vi "Studienarbeit-Luis-Waldhauser-2023.vi"(8 "error in (no error)":errorcluster) -> (0 "error out":errorcluster)   [LabVIEW 2023]
doc: "Technische Hochschule Nürnberg Georg-Simon Ohm\nAbschlußprüfungen Sommersemester 2021 \nOnline (MS-Teams, 13.3.2021 10.00 Uhr - 15.00 Uhr)\nPrüfer: Herbert Pichlik \nZweitkorrektor: Prof. Dr. Michael Chowanetz\n\nNachname: Müller\nVorname: Stefan\nMatrikelnummer: 08154711\n\nHiermit nehme verbindlich an folgenden Prüfungen teil:\n\nWahlpflichtfach: 080efi:WPF:EFI:0 Titel: LabVIEW und Virtuelle Instrumente\n\nWahlfach: 1010:WF:EFI:0 Titel: LabVIEW Vertiefung"
uses:
  <vilib>/Utility/error.llb/DialogType.ctl
  Users/luisw/Downloads/Studiarbeit/Studiarbeit/state.ctl
  <vilib>/event_ctls.llb/eventvkey.ctl
  <vilib>/Utility/NIReport.llb/Report Type.ctl
  <vilib>/Analysis/baseanly.llb/Mean (DBL).vi
  <vilib>/measure/matone.llb/Harmonic Distortion Analyzer 1 Chan.vi
  <vilib>/measure/maspectr.llb/FFT Power Spectrum and PSD for 1 Chan.vi
  <vilib>/printing/OpenHTMLReport.llb/Open HTML Report in Browser (Path).vi
  <vilib>/Utility/NIReport.llb/NI_report.lvclass
  <vilib>/Utility/NIReport.llb/NI_ReportGenerationCore.lvlib
  <vilib>/measure/NI_MABase.lvlib
  <vilib>/measure/NI_MAPro.lvlib
  <vilib>/Analysis/NI_AALBase.lvlib
panel:
  out "path out":path
  out "Time":string="09:57:22"
  out "Date":string="12.03.2021"
  in  "Tab Control":enum32{"GUI", "Input", "Hidden", "Admin"}(tab)
  out "Sequence Comment":string
  out "Name":string
  out "Seq Measurement":T1(array[cluster])
  in  "Load Sequence":path=path "C:/Program Files/National Instruments/LabVIEW 2020/user.lib/SoSe2021/Sequence-01.xlsx"
  out "FFT":cluster{"f0":dbl, "df":dbl, "magnitude":dbl[]}(graph)={"f0"=0.0, "df"=1.0, "magnitude"=[2.6327073338101692e-05, 4.327304114792483e-05, 1.5673481931988e-05, 0.00025407252568578504, 0.0006345873730570163, 0.001098990914477157, 0.0008159585478017789, 1.2611184277899417, 5.146224925426655, 1.3095648931593402, 2.63970380788412e-05, 0.0006386317455637907, 0.0012590716223286752, 0.0005410344712417312, 0.0001693664822519534, 0.0004908339259456577, 0.0011777334761568917, 0.00037163963536089004, 3.021983314851664e-05, 0.00017377346672736057, 0.0003762593897253986, 0.00023256570049066358, 0.00012724272038241313, 0.000178513498907416, 0.00021924620032822906, 0.0001544896302861912, 8.457623674491461e-06, 5.403062950323495e-05, 0.0001296238557588327, 0.00016495018928055702, 0.0003034184772940682, 0.00015646022009288462, 0.00031162575785944626, 0.0012565613166387428, 0.0006107618849779327, 7.515890864872665e-06, 0.0001419118218565884, 8.036975874934862e-05, 8.488687318252203e-05, 2.5141530202907425e-05, 2.673290688424461e-05, 0.00018239018640602903, 0.0005477270664906835, 0.0014690375427782237, 0.0005559107924960337, 8.301140037468495e-05, 0.00012101523160707916, 0.0008051848168213473, 0.0006343845922274333, 1.3569945226961809e-05, 0.0002627792110390153, 0.0002406122221775621, 0.0002163088212400089, 0.0005756861353742484, 0.0006540662987181892, 0.0005760057147609353, 0.001168214064104931, 0.0009142393249436326, 3.7459985637611555e-05, 6.58826949190464e-05, 0.0003019406937540107, 0.00018554779716880925, 9.112019612896804e-05, 0.0002658304606239494, 0.0005842272847474148, 0.001822778790135895, 0.0020011462573474594, 0.000770952197268878, 0.0003802029039891558, 2.1515126635341356e-05, 8.549323495065751e-05, 4.6310151827152625e-05, 9.24162402997269e-05, 7.024420564693392e-05, 0.00020170519648798685, 0.0008603793021965292, 0.0008822311938917643, 0.001716853456240963, 0.00039036674041830654, 0.0006307930109717719, 0.002044627565204085, 0.0011767234719083748, 0.00020159725845851647, 7.759760038327143e-05, 0.0007509384980458659, 0.0002221474003132149, 0.00016765791243669574, 6.896494488849775e-05, 2.992435621102185e-05, 0.0001591877555499712, 0.0006627411738638841, 0.0006823777206984923, 0.00015280161807136624, 4.9723659888706556e-05, 0.00015953763055465215, 0.00021839526016487058, 6.904122739035353e-05, 0.0003228624565004558, 0.0008641263395326468, 0.0004885756306196472, 5.5452575762701354e-05, 6.667888896910418e-05, 0.00016195387231479331, 0.0005157262849646858, 0.00018487779477048604, 0.0005163607105677836, 0.0008405910681775814, 9.914286246284125e-05, 0.0003983930841559924, 0.0006755226388984388, 1.557357874689003e-05, 3.5271995415016136e-06, 0.00011873017943008137, 0.0001178216082098147, 0.0003321531164868442, 0.0002823966252785709, 0.0001271820869068118, 0.00015734413774907115, 0.00011336787749456681, 0.00030849395695113554, 0.0012548186928315786, 0.0009022685720360012, 5.297998902547502e-05, 2.3303881834746823e-05, 0.00022979277121929284, 9.992147446179476e-05, 0.00014219787549692135, 0.00036985584741512086, 0.0005451942969393532, 0.00022508503372422933, 0.0010284913682260671, 0.0013684067307147309, 0.0004522588358697734, 0.0002703600366179861, 5.5588453885048256e-05, 1.587439002785841e-05, 0.00011966475460832903, 0.00010662390359710843, 9.529947631894765e-05, 9.900928679592479e-05, 0.0007085109743305238, 0.00020493016828895114, 3.9234127841945937e-05, 5.8382921609386196e-05, 6.74673457346776e-05, 3.1706979194275405e-05, 5.5114477174054164e-05, 4.1244190248820976e-05, 8.318994464694256e-05, 0.00021409167282633557, 7.076373237749193e-05, 0.0004444126722076365, 1.4431314640259825e-05, 0.0003017498107005694, 0.00019778188880576763, 0.0004790860486344645, 0.0006681849923944, 0.0005240711139280371, 0.0002346300453842311, 0.0002079119924688067, 0.00014490709524552807, 0.00013212635076267408, 9.022508495594329e-05, 0.000330333713353353, 4.280470532497084e-06, 0.00010134846466738688, 2.400909755508234e-05, 0.00010985927008078305, 0.0003929981111498782, 0.0005400793749820781, 0.0004520034503300079, 9.17009482877119e-05, 0.00011737238653380866, 0.00010319090589896972, 1.6439537841938072e-06, 0.0001283612831574683, 0.00028905567066825236, 0.00021147750147839086, 2.04220484868536e-05, 8.465208277084334e-05, 3.623808768161366e-05, 0.0003773213469952989, 0.00012937830574505138, 0.0003866640298215692, 7.132733306923889e-05, 5.2771987655576355e-05, 5.4455648893278534e-06, 5.582730151819657e-05, 0.00014251337916616028, 0.000289780881654889, 0.0004561705450740981, 0.00038478215089753705, 0.0002210077831533168, 0.0007471071677454081, 0.0003449876614190816, 0.00017098320919503408, 0.0001627782782032192, 5.407709388274651e-05, 8.118267267911216e-05, 0.0003582112784618244, 0.0001058911842660299, 0.00014764686268978913, 0.0006102098596987694, 0.0010224941269298374, 0.0006142769875164898, 2.429043677273379e-05, 0.00020167799747654433, 0.00027349153731283285, 0.00010652987123481969, 0.00047708623255439294, 0.0002835863321248803, 0.00022666555138427813, 0.00018751311544084294, 0.0005025289156892825, 0.0005513325910197092, 0.00015378064696769248, 0.0002673977071019374, 0.001265710465499206, 0.0012525023560171226, 0.0005583816477007426, 0.0010473831905999306, 0.0004138865662840121, 0.00047661363730101494, 0.00036919758526177354, 0.0005556972807035322, 0.00034985399709021667, 7.227856284505558e-05, 2.484248564915029e-05, 0.0002593530873531126, 0.0004305355264604284, 0.00026718205836529684, 1.170364600771437e-05, 9.081409533965501e-05, 0.0004154949313148937, 0.00015867291693487002, 0.0006748746734591998, 0.0017578373986235508, 0.0011278285368419264, 0.00046422596107479556, 0.00027962023594540824, 0.0005775526760640319, 0.000348737429386306, 7.683788097177486e-05, 0.0002936022822418179, 0.00030606360872103183, 0.0002660397004358208, 0.0002511983013672862, 0.00022195748812371563, 2.6812320443664388e-05, 0.0004652622263041534, 0.00040144699917068853, 0.0005318184387495809, 0.0012292959696925026, 0.0007158581677641183, 0.00015573498368878547, 0.00036763553761812504, 0.0007452008248718833, 0.0002088236321531605, 0.00010044280294584974, 8.768864059720181e-05, 0.0011104239970920605, 0.0009714569717405014, 0.00012478845574850057, 0.0002896022872338543, 0.00011380260511792134, 0.00011609365864049848, 0.0001645627835783424, 8.273302020755056e-06, 0.0001273923338862413, 0.00012192135645917483, 0.0006458957658063327, 0.001961624503777706, 0.0008683685881627775, 0.0004032281838636848, 0.000548147657478664, 0.00031638587226378375, 0.00012466244576232727, 8.838079592266715e-05, 0.00043460312842646644, 0.0003834237828468636, 0.00037316912856644695, 0.00060344395818078, 1.683531145123034e-05, 0.00030568713365733527, 0.0002315984371667084, 0.00034349875239446614, 0.00029668893138926284, 0.00013204165559261582, 0.00017675503737417739, 0.00041309657840596305, 0.0006184943307073788, 0.0008145268456990111, 0.0005649691133920281, 6.785328288155477e-05, 0.00020536530337127073, 0.0005863178094299846, 0.00027736649921717137, 0.00016780002735215257, 0.00019302759514753238, 5.063732917744958e-05, 6.747026032270585e-05, 0.00012296782407189121, 0.00012680484627711336, 4.017049045582695e-05, 1.0542002602779412e-05, 0.00015140447626373743, 0.0003270763360628557, 0.0009132076728721379, 0.0007117321320466275, 0.0002701070497460904, 7.767786860327002e-05, 0.0004127685891342999, 0.0007593140526463135, 0.00014603985824328074, 1.839588768548391e-05, 8.854903396651383e-05, 0.001510074954756099, 0.0014970433822190815, 0.00022377171634273968, 7.40078778780655e-05, 0.0001260163274678509, 0.0002690832346931617, 0.00018954397390870325, 0.00012028589539187629, 0.0004420355166061732, 0.0004304822596218248, 0.00010638307132800972, 0.00034854574449151414, 0.0004748708843077739, 0.0005232055780611728, 0.00024104491309061724, 6.550599619929381e-05, 0.0001967571133864732, 0.001690127224118065, 0.0012191715839013064, 0.0006238581848276428, 0.00021329110677481338, 1.8724545776554444e-06, 5.57716885110554e-05, 0.00046073282714765017, 0.0005326566757684097, 1.4265211641909113e-05, 0.0005711315473369955, 0.0002463747479256263, 0.0005206890545715398, 0.0005383562038977527, 0.0001792375943564807, 7.569313172701478e-06, 0.0002943537228089917, 0.00030056992668579916, 0.0004986944194498144, 0.0003126687463058902, 1.7233215897759166e-05, 5.950439167688006e-05, 0.00011063406782657094, 0.0010036306046102765, 0.0011349924930043095, 0.00020808221373166372, 6.0812862217454125e-05, 0.0002528431513787704, 0.00018560876652507532, 0.00011056547080725772, 4.847841127827966e-05, 0.00019744320370588126, 9.946560937693087e-06, 1.78371354895216e-05, 9.607045175266706e-05, 0.0004663533026559159, 0.0001423982837765148, 0.00010181978712883213, 0.0005963237754031276, 0.0004147550451140529, 7.50474189184072e-05, 0.00011012376636404323, 0.00021285367807187213, 0.00019556163753912487, 8.23505460985615e-05, 0.0008061851705744255, 0.0006564639754021919, 0.00015642536696461196, 0.000288092132758149, 0.0006433508370270708, 0.00018978462822871446, 0.0002497515782830022, 7.204422289863458e-05, 0.0004085327441515991, 0.0006028559577958507, 0.00011644163681742595, 0.0008403758616763091, 0.0005214119761935168, 0.00089871247291811, 0.0008856869691431593, 0.0008573507042331388, 0.0007502672075876003, 0.0004355395938557245, 1.2181465117333604e-05, 0.0003647099505578123, 0.0004663709650943618, 0.00012010027467200875, 2.8713980945845295e-05, 0.0003940146282055314, 0.00046910276251854857, 0.0014652163284750008, 0.0017714139117713068, 0.0005465103305168458, 6.425632728723554e-05, 0.00012988992696625823, 0.0006308834370315849, 0.00012961752910184627, 0.0003576845332009546, 0.0005942435003096243, 0.00047235272020075927, 0.00019032673048730492, 0.00032843871184392014, 0.0005687728242438977, 0.0005558290709883292, 0.0003021026755876742, 0.00016265338264041522, 0.00012779644566021477, 9.927143887443357e-06, 0.00012036335148449488, 4.024603492691524e-05, 0.000358560336537118, 0.0008602402790443771, 0.00020220124847786388, 0.00011683033349866944, 0.00025808388099077056, 0.0003138609923650052, 0.00014613220543453398, 9.91159807304533e-05, 0.00024484808696432456, 7.479331028947645e-05, 3.937996877771911e-05, 0.00016609254992539353, 0.00026281509128464375, 0.00022488247973952882, 1.048968003988041e-05, 0.0002252322962697982, 9.959590330233384e-06, 0.0003922086595653612, 4.7099927447452256e-05, 0.0004412965429839095, 4.354706962513962e-05, 0.0001343021921939159, 0.0002362328219880965, 7.049057860101398e-05, 3.583451109915395e-05, 3.32302384477848e-05, 0.0003412923472488345, 0.00013171171221900988, 0.00010614858513008197, 0.00046452570350281744, 0.0009337626187577811, 0.0009240917284625516, 0.0008198839260292418, 0.0006269376741399117, 0.00037747479356341765, 0.000858611421143469, 0.00019196150254664442, 5.8408259860901346e-05, 0.00041826024652877347, 0.0004652633308654851, 0.00030277470437015277, 0.00010310684292206175, 0.0002811495292953991, 6.305363857177877e-05, 0.00023032675798953793, 0.00027552138522875556, 9.823955313469193e-05, 0.0007328700729269113, 0.0002749869408836214, 1.682175072600851e-05, 0.0001421520316393631, 0.00010501740939574318, 5.477993711745696e-05, 7.34163423624223e-05, 0.000193109453558897, 0.0002894475707541855, 2.8212722527595225e-05, 0.0004719394826000178, 0.00012237020293320028, 0.0006059216525190111, 0.0002461198656164835, 0.0010126400496228327, 0.0002958263229237784, 4.5478851643752225e-05, 0.00016853484247170586, 0.0002639936035976632, 8.337357594227231e-05, 0.00016432445954141272, 8.900407902992552e-05, 0.0002710155341272003, 0.00012959083585887182, 0.0007030202011662352, 6.942812932076818e-05, 0.000371195311615697, 0.001400583850123373, 0.0012881195999427772, 0.0009540615706532982, 0.0005821178019752567]}
  out "Transaction":string="Shutdown"
  in  "Resume":bool
  out "Halted?":bool
  in  "Halt":bool
  in  "stop":bool=TRUE
  out "Timesignal":waveform(dbl)(graph)={"t0"=timestamp(14.0 s since 1904-01-01), "dt"=0.001, "Y"=array[1000 elements]}
  in  "Start":bool
  out "Waveform":string
  out "Max Value":dbl
  out "Min Value":dbl
  out "Mean Value":dbl format="%0.2f"
  out "Amplitude":dbl
  out "Frequency":dbl
  out "Noise Level":dbl
  out "THD Value":dbl format="%.2p"
  out "THD Calculated":dbl[](array[numeric])=[0.03975861998712104, 0.12184614595401447, 0.6874588867791076, 0.4483840550739134, 0.7933340252119325, 0.09551189336771507, 0.16365956881088106, 0.6266336784336342, 0.7816349376414278, 0.4562491842624781, 0.12793609131885555, 0.02750744215155403, 0.44691834586275686, 0.7822373702923411, 0.051916156114339106]
  out "THD Exceeded":bool[](array[boolean])
  in  "Sequence Measurement Input":T1(array[cluster]) {"THD_Limit" min=0.0 max=1.0 step=0.01; "Noise" min=0.0 max=10.0 step=0.1; "Frequency" min=0.0 max=1000.0 step=1.0; "Amplitude" min=0.0 max=10.0 step=0.1}
  in  "Save Sequence":bool
  in  "User":string
  in  "Comment":string
  out "Sequence File":string
  out "General_Info":T2
  out "Loq_Seq 2":T3(array[cluster])
  out "Sequence_File":path
  out "Time":string[](array[string])=["09:54:06", "09:54:07", "09:54:08", "09:54:09", "09:54:10", "09:54:11", "09:54:12", "09:54:13", "09:54:14", "09:54:15", "09:54:16", "09:54:17", "09:54:18", "09:54:19", "09:54:20"]
  out "MAX":dbl[](array[numeric])=[2.27393051244096, 5.0392142809948925, 7.7948229991906555, 10.994167680455824, 4.417238946374613, 8.081222408397412, 4.938759913961892, 2.998128719739788, 0.9911050409919856, 1.6994539558744703, 2.249828084878313, 4.358791189496003, 3.19526859777135, 3.674559787768871, 3.7780461747537277]
  out "MIN":dbl[](array[numeric])=[-2.2840724232625, -5.041632709827746, -7.796728883881844, -10.99766945322614, -4.577880852035904, -8.124820044291972, -4.746638854079128, -2.9998631493133003, -0.9909090993690596, -1.6975713331601046, -2.1999025738510065, -4.360441249435146, -3.1941613240887374, -3.6354160522071917, -3.787730730606972]
  out "MEAN":dbl[](array[numeric])=[0.1156993772066776, -0.0008635806207144958, -0.012725991993728331, -0.012883347191881079, 0.03397443373431783, 0.053108227883207584, 0.020494035280072383, 0.04242488943858582, 5.295077057532216e-05, -0.002016744784994759, -0.0011573976155003732, -0.0018931501032122453, 0.013541189971497499, -0.03334461529697598, -0.0028203900025636375]
  out "THD":dbl[](array[numeric])=[0.03975861998712104, 0.12184614595401447, 0.6874588867791076, 0.4483840550739134, 0.7933340252119325, 0.09551189336771507, 0.16365956881088106, 0.6266336784336342, 0.7816349376414278, 0.4562491842624781, 0.12793609131885555, 0.02750744215155403, 0.44691834586275686, 0.7822373702923411, 0.051916156114339106]
  out "Freq":dbl[](array[numeric])
  out "Amp":dbl[](array[numeric])
  out "Noise":dbl[](array[numeric])
  out "Numerics":dbl[][](array[numeric])
  out "Waveforms":string[](array[string])
  out "Time+Waveform":string[][](array[string])
  # "Studienarbeit Luis Waldhauser"
  # "Waveform         Amplitude       Frequency        Noise          THD Limit            Teststep Name"
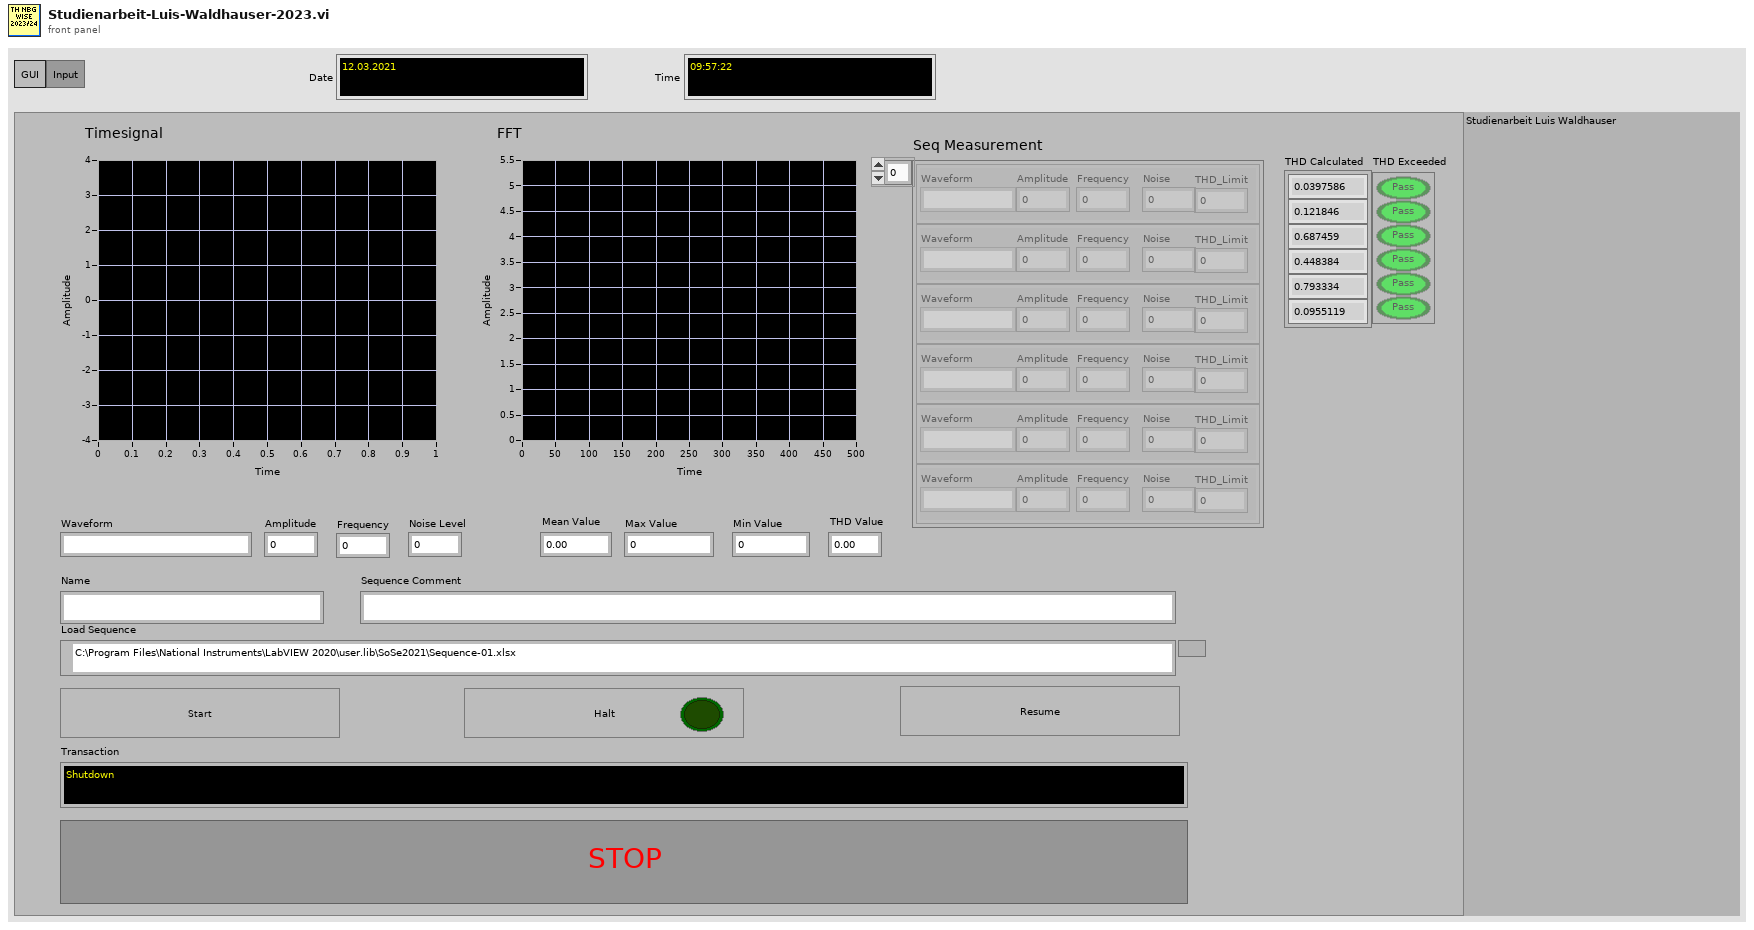
[diagram p1: front panel]
types:
  T1 = cluster{"Waveform":enum16{"", "Sine Wave", "Triangle Wave", "Square Wave", "Sawtooth Wave"}, "Amplitude":dbl, "Frequency":dbl, "Noise":dbl, "THD_Limit":dbl, "Teststep_Name":string}[]
  T2 = cluster{"User":string, "Comment":string, "Date":string, "Time":string, "Sequence_File":path}
  T3 = cluster{"Waveform":i32, "Teststep_Name":string, "Amplitude":dbl, "Frequency":dbl, "Noise":dbl, "THD_Limit":dbl, "THD_Calculated":dbl, "THD_Exceeded":bool, "Timesignal":waveform(dbl), "FFT":cluster{"f0":dbl, "df":dbl, "magnitude":dbl[]}}[]
  T4 = typedef "state.ctl" = enum16{"Initialize", "Process", "Report", "Halt", "Shutdown"}
  T5 = typedef "eventvkey.ctl" = enum16{"ASCII", "Enter", "Return", "Shift", "Ctrl", "Alt", "Cmd", "Opt", "Caps", "NumLock", "Clear", "Break", "Up", "Down", "Left", "Right", "Insert", "Delete", "Home", "End", "PageUp", "PageDown", "Escape", "Help", "Pause", "ScrollLock", "F1", "F2", "F3", "F4", "F5", "F6", "F7", "F8", "F9", "F10", "F11", "F12", "F13", "F14", "F15", "F16", "F17", "F18", "F19", "F20", "F21", "F22", "F23", "F24", "Play", "VolumeUp", "VolumeDown", "Mute", "Two Byte Char"}
  T6 = cluster{"Waveform":i32, "Teststep_Name":string, "Amplitude":dbl, "Frequency":dbl, "Noise":dbl, "THD_Limit":dbl, "THD_Calculated":dbl, "THD_Exceeded":bool, "Timesignal":waveform(dbl), "FFT":cluster{"f0":dbl, "df":dbl, "magnitude":dbl[]}}
  T7 = enum16{"Sine Wave", "Triangle Wave", "Square Wave", "Sawtooth Wave"}
  T8 = typedef "NI_ReportGenerationCore.lvlib/Report Type.ctl" = enum16{"HTML", "Word", "Excel"}
  T9 = typedef "DialogType.ctl" = u16
  T10 = enum16{"", "Sine Wave", "Triangle Wave", "Square Wave", "Sawtooth Wave"}
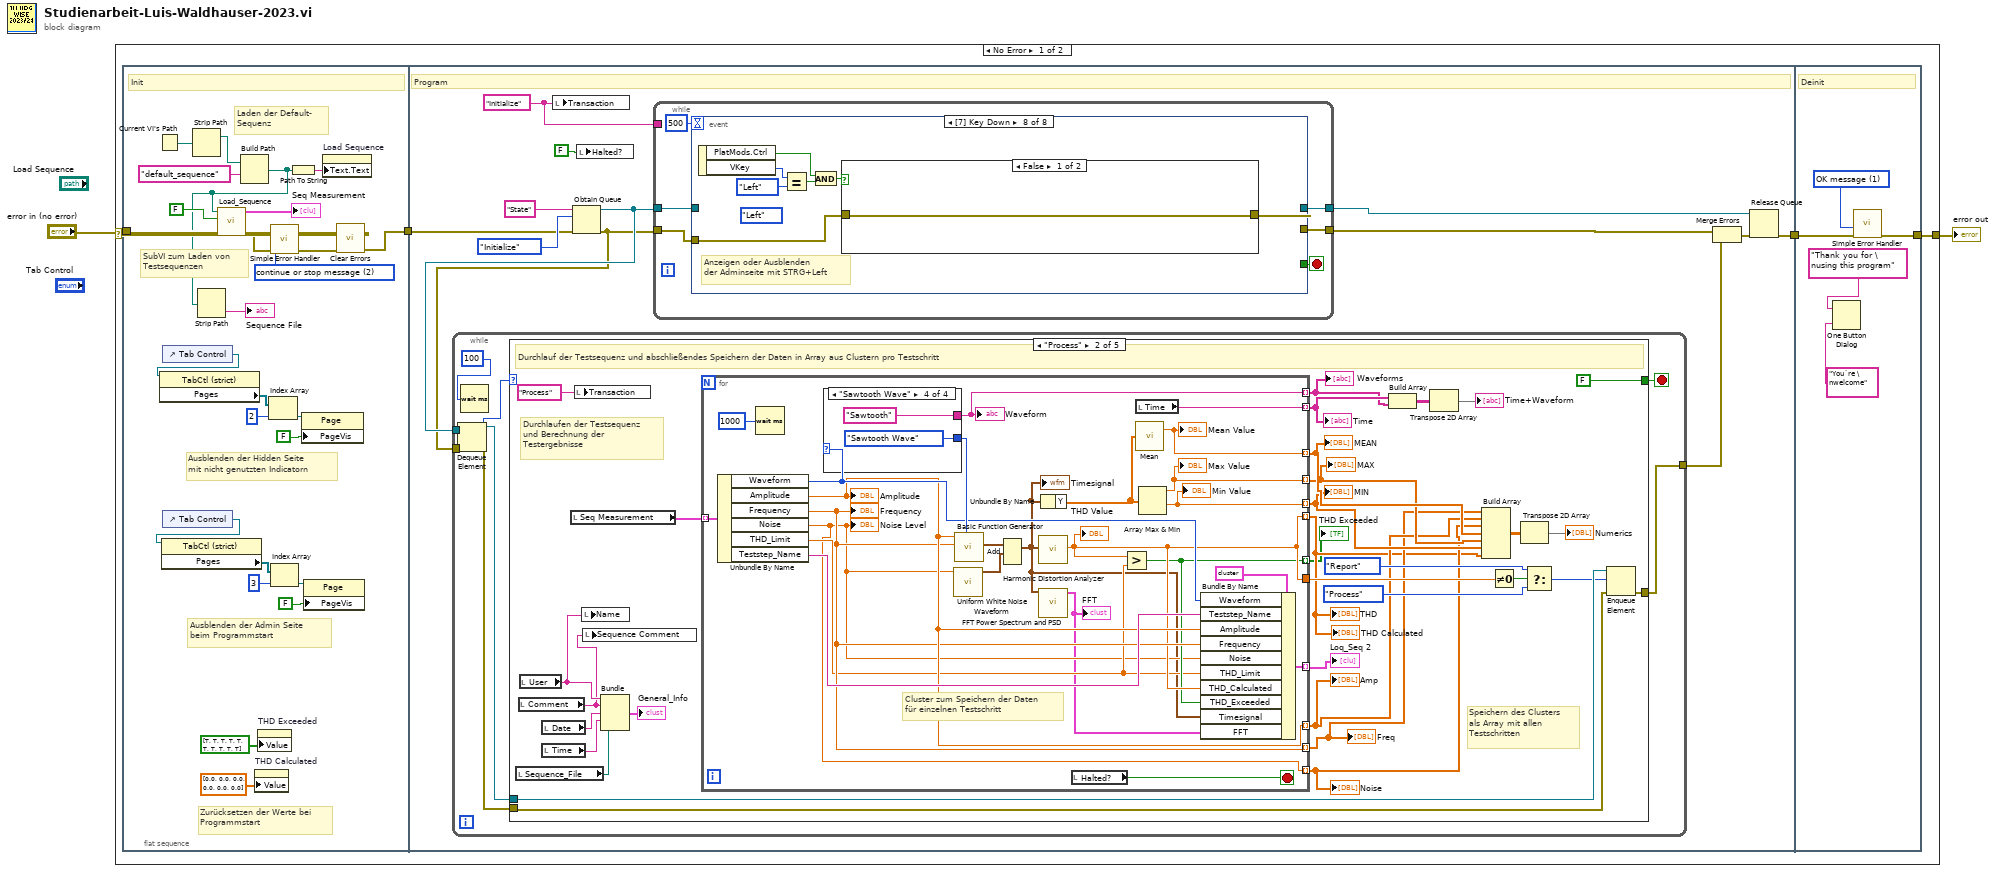
[diagram p0: block diagram]
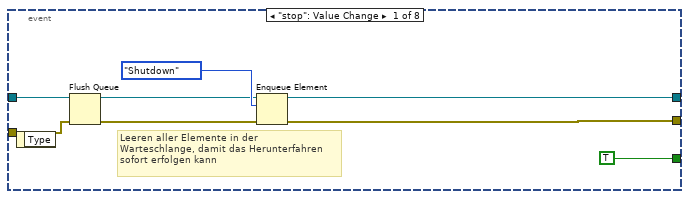
[diagram p2: hidden frame]
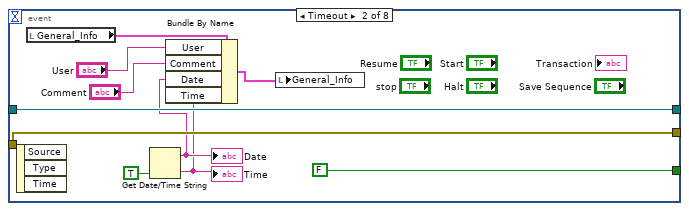
[diagram p3: hidden frame]
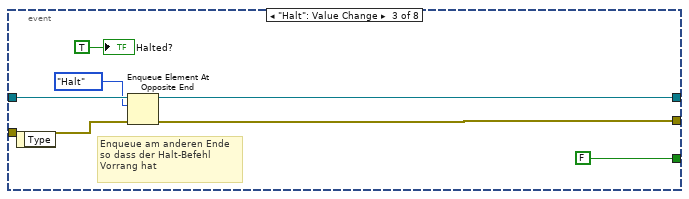
[diagram p4: hidden frame]
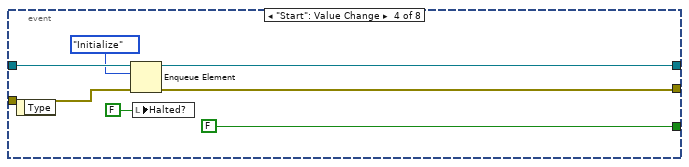
[diagram p5: hidden frame]
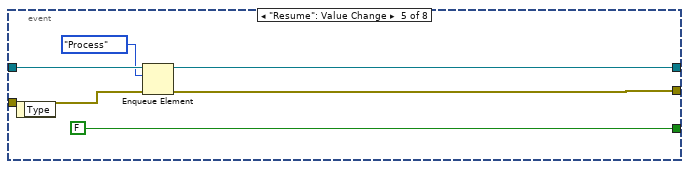
[diagram p6: hidden frame]
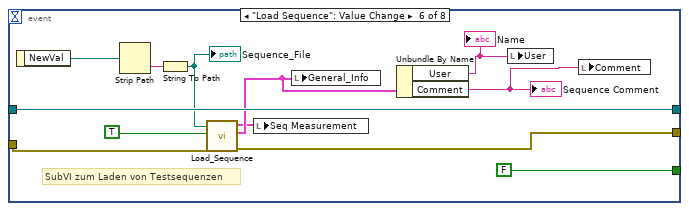
[diagram p7: hidden frame]
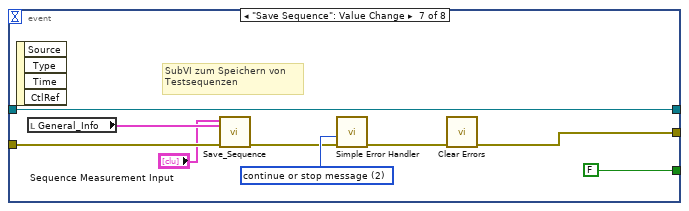
[diagram p8: hidden frame]
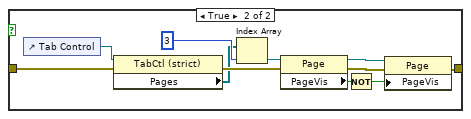
[diagram p9: hidden frame]
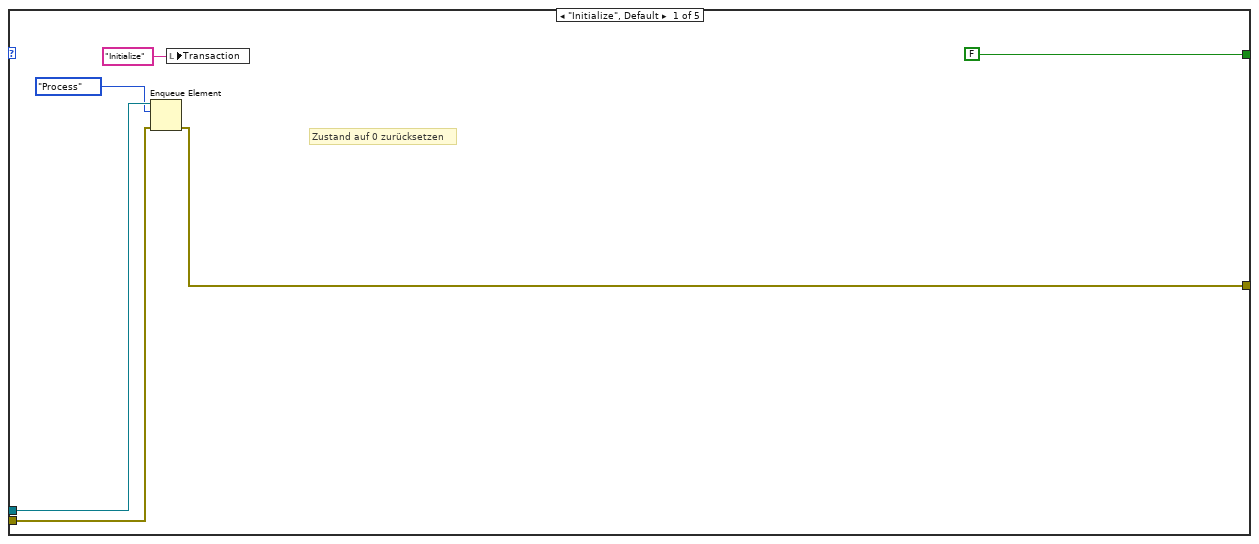
[diagram p10: hidden frame]
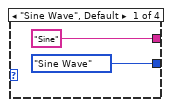
[diagram p11: hidden frame]
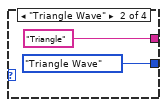
[diagram p12: hidden frame]
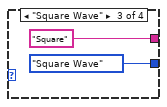
[diagram p13: hidden frame]
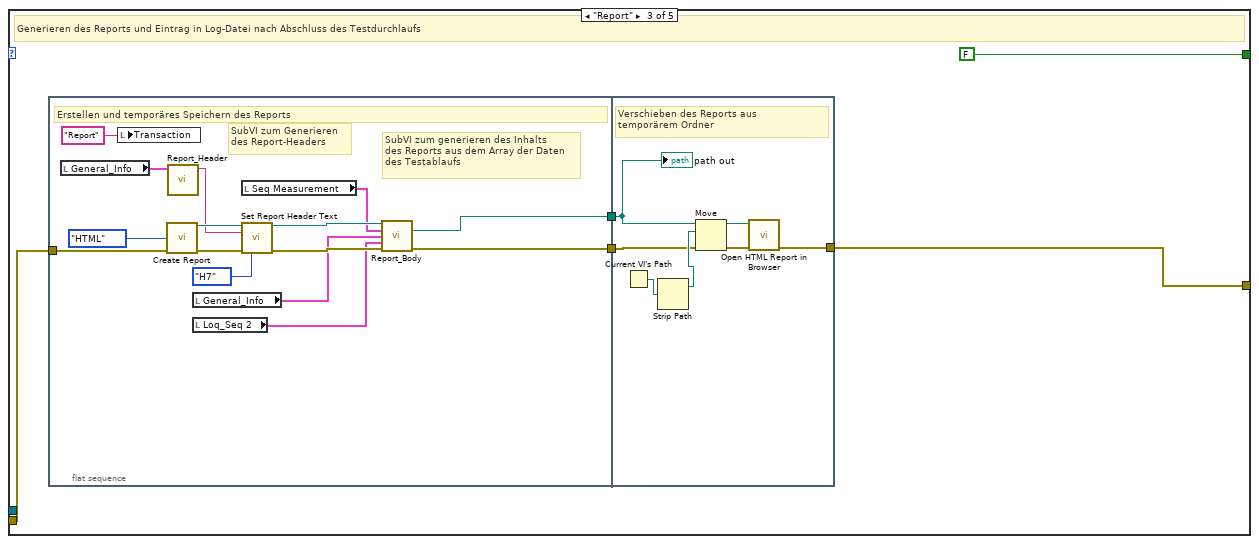
[diagram p14: hidden frame]
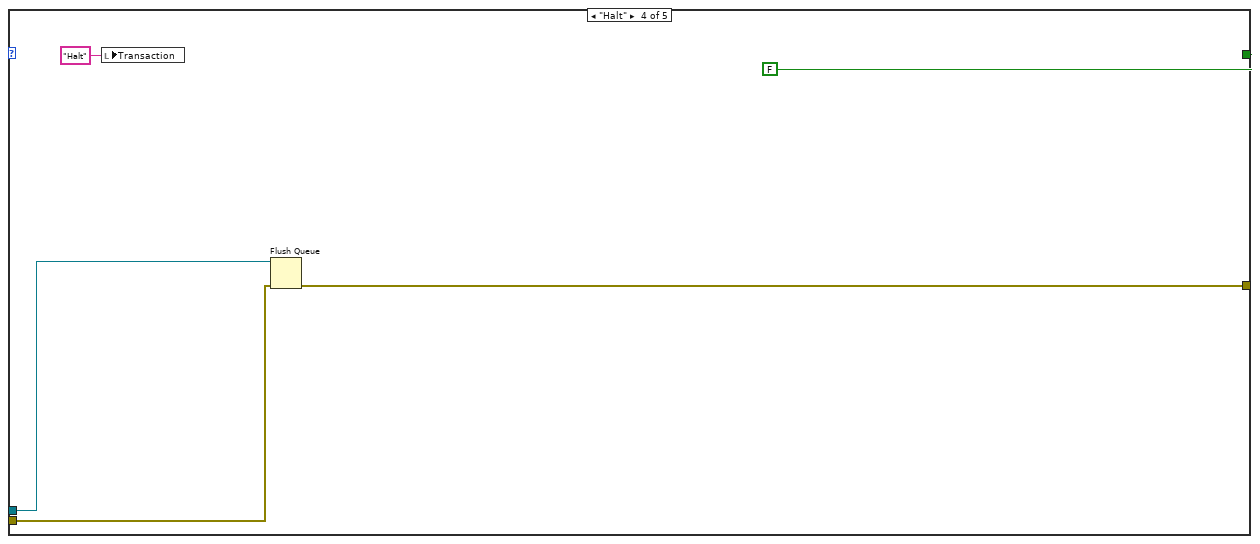
[diagram p15: hidden frame]
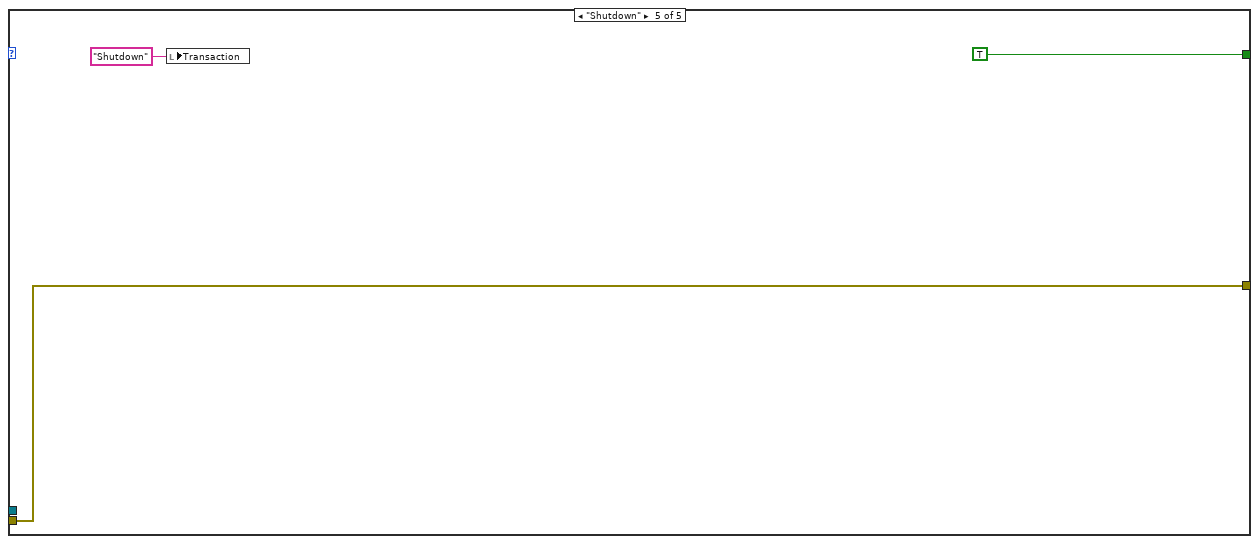
[diagram p16: hidden frame]
diagram:
  n1 = case shown="No Error" "error in (no error)" {
    selector: "error in (no error)" -> [w6 w246]
    tunnel: [w3 w246] -> w1
    frame No Error {
      n2 = flat-sequence {
        tunnel: w6 -> [w31]
        tunnel: [w8] -> w5
        tunnel: w5 -> [w33]
        tunnel: [w32] -> w4
        tunnel: w4 -> [w245]
        tunnel: [w244] -> w3
        frame #0 {
          w7 = T9 2 items=["no dialog", "OK message", "continue or stop message", "OK message + warnings", "continue/stop + warnings"] ("type of dialog (OK msg:1)")
          # "Laden der Default-\nSequenz"
          # "Ausblenden der Admin Seite \nbeim Programmstart"
          # "Zurücksetzen der Werte bei\nProgrammstart"
          # "Ausblenden der Hidden Seite\nmit nicht genutzten Indicatorn"
          # "SubVI zum Laden von\nTestsequenzen"
          # "Init"
          n3 = Current VI's Path() -> (path=w15:path)
          n4 = control-ref of="Tab Control"() -> (w26:refnum<vi>)
          n5 = property class="TabCtl (strict)"(reference=w26) -> ("Pages"=w25:refnum<vi>[])  [unwired: 1 in, 2 out]
          n6 = control-ref of="Tab Control"() -> (w16:refnum<vi>)
          n7 = property class="TabCtl (strict)"(reference=w16) -> ("Pages"=w18:refnum<vi>[])  [unwired: 1 in, 2 out]
          n8 = Strip Path(path=w15) -> (stripped path=w13:path)  [unwired: 1 out]
          n9 = Build Path(base path=w13, name or relative path="default_sequence" ("string")) -> (appended path=w11:path)
          n10 = Strip Path(path=w11) -> (name=→"Sequence File":string)  [unwired: 1 out]
          n11 = call "Load_Sequence.vi"("error in (no error)"=w31, "relative Path"=FALSE, "Path"=w11) -> ("error out"=w10:errorcluster, "Seq_Measurement"=→"Seq Measurement":T1)  [unwired: 6 in, 1 out]
          n12 = property on="THD Calculated" class="Arr (strict)"("Value"=dbl[] [0.0, 0.0, 0.0, 0.0, 0.0, 0.0] ("THD_Calculated")) -> ()  [unwired: 2 in, 2 out]
          n13 = property on="THD Exceeded" class="Arr (strict)"("Value"=bool[] [TRUE, TRUE, TRUE, TRUE, TRUE, TRUE, TRUE, TRUE, TRUE, TRUE] ("THD_Exceeded")) -> ()  [unwired: 2 in, 2 out]
          n14 = Index Array(array=w25, index=2) -> (element=w24:refnum<vi>)
          n15 = call <vilib>:"Simple Error Handler.vi"("type of dialog (OK msg:1)"=w7, "error in (no error)"=w10) -> ("error out"=w9:errorcluster)  [unwired: 3 in, 4 out]
          n16 = Index Array(array=w18, index=3) -> (element=w19:refnum<vi>)
          n17 = Path To String(path=w11) -> (string=w12:string)
          n18 = property class="Page"(reference=w24, "PageVis"=FALSE) -> ()  [unwired: 1 in, 2 out]
          n19 = property class="Page"(reference=w19, "PageVis"=FALSE) -> ()  [unwired: 1 in, 2 out]
          n20 = property on="Load Sequence" class="Path"("Text.Text"=w12) -> ()  [unwired: 2 in, 2 out]
          n21 = call <vilib>:"Clear Errors.vi"("error in (no error)"=w9) -> ("error out"=w8:errorcluster)  [unwired: 5 in, 1 out]
        }
        frame #1 {
          w35 = "Initialize" ("Transaction")
          # "Program"
          n22 = local write "Transaction"(w35) -> ()
          n23 = Obtain Queue(name (unnamed)="State", element data type=state."Initialize" ("State Selector"), error in (no error)=w33) -> (queue out=w41:refnum<queue>, error out=w40:errorcluster)  [unwired: 2 in, 1 out]
          n24 = while {
            tunnel: w41 -> [w135]
            tunnel: w40 -> [w134]
            tunnel: [w128] -> w38
            stop <- w132 stop-if-true
            n25 = Dequeue Element(queue=w135, error in (no error)=w134) -> (queue out=w130:refnum<queue>, element=w133:T4, error out=w131:errorcluster)  [unwired: 1 in, 1 out]
            n26 = Wait (ms)(milliseconds to wait=u32 100) -> ()  [unwired: 1 out]
            n27 = case shown="\"Process\"" w133 {
              tunnel: [FALSE FALSE FALSE FALSE TRUE] -> w132
              tunnel: w131 -> [w140 w172 w209 w236 w239]
              tunnel: w130 -> [w139 w173 _ w237 _]
              tunnel: [w137 w167 w208 w234 w239] -> w128
              frame "Initialize", Default {
                # "Zustand auf 0 zurücksetzen"
                n28 = Enqueue Element(queue=w139, element=state."Process" ("State Selector"), error in (no error)=w140) -> (error out=w137:errorcluster)  [unwired: 1 in, 2 out]
                n29 = local write "Transaction"("Initialize" ("Transaction")) -> ()
              }
              frame "Process" {
                # "Speichern des Clusters\nals Array mit allen \nTestschritten"
                # "Durchlaufen der Testsequenz\nund Berechnung der \nTestergebnisse"
                # "Durchlauf der Testsequenz und abschließendes Speichern der Daten in Array aus Clustern pro Testschritt"
                n30 = local read "Sequence_File"() -> (w145:path)
                n31 = local read "Comment"() -> (w142:string)
                n32 = local read "User"() -> (w143:string)
                n33 = local read "Date"() -> (w147:string)
                n34 = local read "Time"() -> (w146:string)
                n35 = local read "Seq Measurement"() -> (w154:T1)
                n36 = local write "Transaction"("Process" ("Transaction")) -> ()
                n37 = local write "Name"(w143) -> ()
                n38 = local write "Sequence Comment"(w142) -> ()
                n39 = Bundle("User"=w143, "Comment"=w142, "Date"=w147, "Time"=w146, "Sequence_File"=w145) -> (→"General_Info":T2)  [unwired: 1 in]
                n40 = for {
                  tunnel: [w180] -> w150 mode=indexing
                  tunnel: [w180] -> w165
                  tunnel: [w193] -> w157 mode=indexing
                  tunnel: [w192] -> w156 mode=indexing
                  tunnel: [w190] -> w158 mode=indexing
                  tunnel: [w189] -> w163 mode=indexing
                  tunnel: [w188] -> w162 mode=indexing
                  tunnel: [w181] -> w152 mode=indexing
                  tunnel: [w182] -> w153 mode=indexing
                  tunnel: [w176] -> w151 mode=indexing
                  tunnel: w154 -> [w187] mode=indexing
                  tunnel: [w179] -> w149 mode=indexing
                  tunnel: [w178] -> w148 mode=indexing
                  stop <- w194 stop-if-true
                  # "Cluster zum Speichern der Daten\nfür einzelnen Testschritt"
                  n41 = Unbundle By Name(w187) -> ("Waveform"=w184:T10, "Amplitude"=w182:dbl, "Frequency"=w181:dbl, "Noise"=w176:dbl, "THD_Limit"=w177:dbl, "Teststep_Name"=w183:string)
                  "Amplitude" <- w182
                  "Frequency" <- w181
                  "Noise Level" <- w176
                  n42 = Wait (ms)(milliseconds to wait=u32 1000) -> ()  [unwired: 1 out]
                  n43 = case shown="\"Sawtooth Wave\"" w184 {
                    tunnel: [T7."Sine Wave" ("signal type") T7."Triangle Wave" ("signal type") T7."Square Wave" ("signal type") T7."Sawtooth Wave" ("signal type")] -> w186
                    tunnel: ["Sine" "Triangle" "Square" "Sawtooth"] -> w188
                    frame "Sine Wave", Default {
                    }
                    frame "Triangle Wave" {
                    }
                    frame "Square Wave" {
                    }
                    frame "Sawtooth Wave" {
                    }
                  }
                  "Waveform" <- w188
                  n44 = call <vilib>:"Uniform White Noise Waveform.vi"("amplitude"=w176) -> ("signal out"=w196:waveform(dbl))  [unwired: 9 in, 1 out]
                  n45 = call <vilib>:"Basic Function Generator.vi"("signal type"=w186, "amplitude"=w181, "frequency"=w182) -> ("signal out"=w197:waveform(dbl))  [unwired: 6 in, 2 out]
                  n46 = Add(1:w196, 2:w197) -> (0:w175:waveform(dbl))  [unwired: 1 in, 1 out]
                  "Timesignal" <- w175
                  n47 = call-poly <vilib>:"Harmonic Distortion Analyzer.vi"("signal in"=w175) -> ("THD"=w180:dbl)  [unwired: 5 in, 5 out]
                  "THD Value" <- w180
                  n48 = call-poly <vilib>:"FFT Power Spectrum and PSD.vi"("time signal"=w175) -> ("Power Spectrum / PSD"=w174:cluster{"f0":dbl, "df":dbl, "magnitude":dbl[]})  [unwired: 7 in, 3 out]
                  "FFT" <- w174
                  n49 = Unbundle By Name(w175) -> ("Y"=w191:dbl[])
                  n50 = local read "Halted?"() -> (w194:bool)
                  n51 = Greater?(x=w180, y=w177) -> (0:w179:bool)
                  n52 = local read "Time"() -> (w189:string)
                  n53 = call-poly <vilib>:"Mean.vi"("X"=w191) -> ("mean"=w190:dbl)  [unwired: 1 out]
                  "Mean Value" <- w190
                  n54 = Array Max & Min(array=w191) -> (max value=w193:dbl, min value=w192:dbl)  [unwired: 2 out]
                  "Max Value" <- w193
                  "Min Value" <- w192
                  n55 = Bundle By Name(cluster=T6 {"Waveform"=0, "Teststep_Name"="", "Amplitude"=0.0, "Frequency"=0.0, "Noise"=0.0, "THD_Limit"=0.0, "THD_Calculated"=0.0, "THD_Exceeded"=TRUE, "Timesignal"={"t0"=timestamp(0 s since 1904-01-01), "dt"=1.0, "Y"=[]}, "FFT"={"f0"=0.0, "df"=1.0, "magnitude"=array[500 elements]}}, "Waveform"=w184, "Teststep_Name"=w183, "Amplitude"=w182, "Frequency"=w181, "Noise"=w176, "THD_Limit"=w177, "THD_Calculated"=w180, "THD_Exceeded"=w179, "Timesignal"=w175, "FFT"=w174) -> (w178:T6)
                }
                "THD" <- w150
                "Time" <- w163
                "MAX" <- w157
                "MIN" <- w156
                "MEAN" <- w158
                "Freq" <- w152
                "Amp" <- w153
                "Noise" <- w151
                "Waveforms" <- w162
                "THD Calculated" <- w150
                "THD Exceeded" <- w149
                "Loq_Seq 2" <- w148
                n56 = Build Array(w163, w162) -> (w161:string[][])
                n57 = Transpose 2D Array(2D array=w161) -> (transposed array=→"Time+Waveform":string[][])
                n58 = Build Array(w152, w153, w151, w158, w157, w156, w150) -> (w159:dbl[][])
                n59 = Not Equal To 0?(x=w165) -> (x != 0?=w164:bool)
                n60 = Transpose 2D Array(2D array=w159) -> (transposed array=→"Numerics":dbl[][])
                n61 = Select(t=state."Report" ("State Selector"), s=w164, f=state."Process" ("State Selector")) -> (s? t:f=w169:T4)
                n62 = Enqueue Element(queue=w173, element=w169, error in (no error)=w172) -> (error out=w167:errorcluster)  [unwired: 1 in, 2 out]
              }
              frame "Report" {
                # "Generieren des Reports und Eintrag in Log-Datei nach Abschluss des Testdurchlaufs"
                n63 = flat-sequence {
                  tunnel: w209 -> [w214]
                  tunnel: [w211] -> w207
                  tunnel: [w215] -> w206
                  tunnel: [w228] -> w208
                  tunnel: w207 -> [w230]
                  tunnel: w206 -> [w227]
                  frame #0 {
                    # "SubVI zum generieren des Inhalts\ndes Reports aus dem Array der Daten\ndes Testablaufs"
                    # "SubVI zum Generieren \ndes Report-Headers"
                    # "Erstellen und temporäres Speichern des Reports"
                    n64 = local read "General_Info"() -> (w220:T2)
                    n65 = local write "Transaction"("Report" ("Transaction")) -> ()
                    n66 = call <vilib>:"Create Report.vi"("report type"=Report_Type."HTML" ("Report Type"), "error in (no error)"=w214) -> ("report out"=w222:refnum<class "NI_report.lvclass">, "error out"=w221:errorcluster)  [unwired: 12 in]
                    n67 = call "Report_Header.vi"("General_Info"=w220) -> ("concatenated string"=w213:string)  [unwired: 9 in, 1 out]
                    n68 = local read "General_Info"() -> (w212:T2)
                    n69 = local read "Loq_Seq 2"() -> (w216:T3)
                    n70 = local read "Seq Measurement"() -> (w217:T1)
                    n71 = call-dynamic "Set Report Header Text.vi"("report in"=w222, "left header text"=w213, "error in (no error)"=w221, "HTML header size"=enum16{"H1", "H2", "H3", "H4", "H5", "H6", "H7"}."H7") -> ("report out"=w219:refnum<class "NI_report.lvclass">, "error out"=w218:errorcluster)  [unwired: 10 in]
                    n72 = call "Report_Body.vi"("report in"=w219, "Seq_Measurement"=w217, "General_Info"=w212, "Log_Seq"=w216, "error in (no error)"=w218) -> ("appended path"=w215:path, "error out"=w211:errorcluster)  [unwired: 9 in]
                  }
                  frame #1 {
                    # "Verschieben des Reports aus \ntemporärem Ordner"
                    n73 = Current VI's Path() -> (path=w232:path)
                    n74 = Strip Path(path=w232) -> (stripped path=w231:path)  [unwired: 1 out]
                    n75 = Move(source path=w227, error in=w230, 10:w231) -> (error out=w229:errorcluster, 3:w226:path)  [unwired: 2 in, 1 out]
                    n76 = call-poly <vilib>:"Open HTML Report in Browser.vi"("path"=w226, "error in (no error)"=w229) -> ("error out"=w228:errorcluster)  [unwired: 12 in, 1 out]
                    "path out" <- w227
                  }
                }
              }
              frame "Halt" {
                n77 = local write "Transaction"("Halt" ("Transaction")) -> ()
                n78 = Flush Queue(queue=w237, error in (no error)=w236) -> (error out=w234:errorcluster)  [unwired: 2 out]
              }
              frame "Shutdown" {
                n79 = local write "Transaction"("Shutdown" ("Transaction")) -> ()
              }
            }
          }
          n80 = local write "Halted?"(FALSE ("Halted?")) -> ()
          n81 = while {
            tunnel: w41 -> [w48]
            tunnel: w40 -> [w47]
            tunnel: [w46] -> w39
            tunnel: [w45] -> w37
            tunnel: w35 -> [_]
            stop <- w49 stop-if-true
            n82 = event shown="[7] Key Down" {
              selector: _ -> [_ _ _ _ _ _ _ _]
              dyn-events: _ -> [_ _ _ _ _ _ _ _]
              timeout: 500 -> [_ _ _ _ _ _ _ _]
              tunnel: [TRUE FALSE FALSE FALSE FALSE FALSE FALSE _] -> w49
              tunnel: w48 -> [w53 w66 w71 w81 w87 w98 w108 _]
              tunnel: w47 -> [w51 w65 w74 w80 w86 w93 w103 w113]
              tunnel: [w55 w66 w72 w78 w84 w98 w108 _] -> w46
              tunnel: [w54 w65 w73 w77 w83 w92 w105 w112] -> w45
              event "stop": Value Change {
                # "Leeren aller Elemente in der\nWarteschlange, damit das Herunterfahren\nsofort erfolgen kann"
                n83 = event-data() -> ()  [unwired: 1 in, 1 out]
                n84 = Flush Queue(queue=w53, error in (no error)=w51) -> (queue out=w52:refnum<queue>, error out=w50:errorcluster)  [unwired: 1 out]
                n85 = Enqueue Element(queue=w52, element=state."Shutdown" ("State Selector"), error in (no error)=w50) -> (queue out=w55:refnum<queue>, error out=w54:errorcluster)  [unwired: 1 in, 1 out]
              }
              event Timeout {
                n86 = event-data() -> ()  [unwired: 1 in, 3 out]
                n87 = local read "General_Info"() -> (w63:T2)
                n88 = Get Date/Time String(want seconds? (F)=TRUE) -> (date string=w60:string, time string=w59:string)  [unwired: 2 in]
                "Date" <- w60
                "Time" <- w59
                n89 = Bundle By Name(cluster=w63, "User"="User", "Comment"="Comment", "Date"=w60, "Time"=w59) -> (w58:T2)
                n90 = local write "General_Info"(w58) -> ()
              }
              event "Halt": Value Change {
                # "Enqueue am anderen Ende\nso dass der Halt-Befehl\nVorrang hat"
                n91 = event-data() -> ()  [unwired: 1 in, 1 out]
                n92 = Enqueue Element At Opposite End(queue=w71, element=state."Halt" ("State Selector"), error in (no error)=w74) -> (queue out=w72:refnum<queue>, error out=w73:errorcluster)  [unwired: 1 in, 1 out]
                "Halted?" <- TRUE ("Halted?")
              }
              event "Start": Value Change {
                n93 = event-data() -> ()  [unwired: 1 in, 1 out]
                n94 = Enqueue Element(queue=w81, element=state."Initialize" ("State Selector"), error in (no error)=w80) -> (queue out=w78:refnum<queue>, error out=w77:errorcluster)  [unwired: 1 in, 1 out]
                n95 = local write "Halted?"(FALSE ("Halted?")) -> ()
              }
              event "Resume": Value Change {
                n96 = event-data() -> ()  [unwired: 1 in, 1 out]
                n97 = Enqueue Element(queue=w87, element=state."Process" ("State Selector"), error in (no error)=w86) -> (queue out=w84:refnum<queue>, error out=w83:errorcluster)  [unwired: 1 in, 1 out]
              }
              event "Load Sequence": Value Change {
                # "SubVI zum Laden von Testsequenzen"
                n98 = event-data() -> ("NewVal"=w97:path)  [unwired: 1 in]
                n99 = Strip Path(path=w97) -> (name=w96:string)  [unwired: 1 out]
                n100 = String To Path(string=w96) -> (path=w95:path)
                "Sequence_File" <- w95
                n101 = call "Load_Sequence.vi"("error in (no error)"=w93, "relative Path"=TRUE, "Path"=w95) -> ("error out"=w92:errorcluster, "General_Info"=w91:T2, "Seq_Measurement"=w90:T1)  [unwired: 6 in]
                n102 = local write "Seq Measurement"(w90) -> ()
                n103 = local write "General_Info"(w91) -> ()
                n104 = Unbundle By Name(w91) -> ("User"=w89:string, "Comment"=w88:string)
                "Name" <- w89
                "Sequence Comment" <- w88
                n105 = local write "User"(w89) -> ()
                n106 = local write "Comment"(w88) -> ()
              }
              event "Save Sequence": Value Change {
                w104 = T9 2 items=["no dialog", "OK message", "continue or stop message", "OK message + warnings", "continue/stop + warnings"] ("type of dialog (OK msg:1)")
                # "SubVI zum Speichern von \nTestsequenzen"
                n107 = event-data() -> ()  [unwired: 1 in, 4 out]
                n108 = local read "General_Info"() -> (w101:T2)
                n109 = call "Save_Sequence.vi"("Edit_Seq_Array_Input"="Sequence Measurement Input", "General_Info"=w101, "error in (no error)"=w103) -> ("error out"=w102:errorcluster)  [unwired: 7 in]
                n110 = call <vilib>:"Simple Error Handler.vi"("type of dialog (OK msg:1)"=w104, "error in (no error)"=w102) -> ("error out"=w106:errorcluster)  [unwired: 3 in, 4 out]
                n111 = call <vilib>:"Clear Errors.vi"("error in (no error)"=w106) -> ("error out"=w105:errorcluster)  [unwired: 5 in, 1 out]
              }
              event Key Down {
                (unwired) eventvkey."Left" ("y")
                # "Anzeigen oder Ausblenden\nder Adminseite mit STRG+Left"
                n112 = event-data() -> ("PlatMods.Ctrl"=w115:bool, "VKey"=w110:T5)  [unwired: 1 in]
                n113 = Equal?(x=w110, y=eventvkey."Left") -> (x = y?=w111:bool)
                n114 = And(x=w115, y=w111) -> (x .and. y?=w114:bool)
                n115 = case shown="False" w114 {
                  tunnel: w113 -> [w116 w126]
                  tunnel: [w116 w121] -> w112
                  frame False {
                  }
                  frame True {
                    n116 = control-ref of="Tab Control"() -> (w127:refnum<vi>)
                    n117 = property class="TabCtl (strict)"(reference=w127, error in=w126) -> (error out=w124:errorcluster, "Pages"=w123:refnum<vi>[])  [unwired: 1 out]
                    n118 = Index Array(array=w123, index=3) -> (element=w122:refnum<vi>)
                    n119 = property class="Page"(reference=w122, error in=w124) -> (reference out=w119:refnum<vi>, error out=w120:errorcluster, "PageVis"=w118:bool)
                    n120 = Not(x=w118) -> (.not. x?=w117:bool)
                    n121 = property class="Page"(reference=w119, error in=w120, "PageVis"=w117) -> (error out=w121:errorcluster)  [unwired: 1 out]
                  }
                }
              }
            }
          }
          n122 = Merge Errors(w37, w38) -> (w36:errorcluster)
          n123 = Release Queue(queue=w39, error in (no error)=w36) -> (error out=w32:errorcluster)  [unwired: 1 in, 2 out]
        }
        frame #2 {
          w243 = T9 1 items=["no dialog", "OK message", "continue or stop message", "OK message + warnings", "continue/stop + warnings"] ("type of dialog (OK msg:1)")
          # "Deinit"
          n124 = One Button Dialog(message="Thank you for \nusing this program", button name ("OK")="You´re \nwelcome") -> ()  [unwired: 1 out]
          n125 = call <vilib>:"Simple Error Handler.vi"("type of dialog (OK msg:1)"=w243, "error in (no error)"=w245) -> ("error out"=w244:errorcluster)  [unwired: 3 in, 4 out]
        }
      }
    }
    frame Error {
    }
  }
  "error out" <- w1
